vi "Timing-Watchdog.vi"(0 "milliseconds to wait":u32=5000, 7 "Watch":bool) -> ()   [LabVIEW 2020]
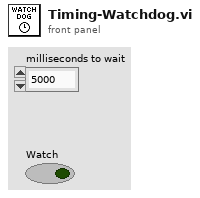
[diagram p1: front panel]
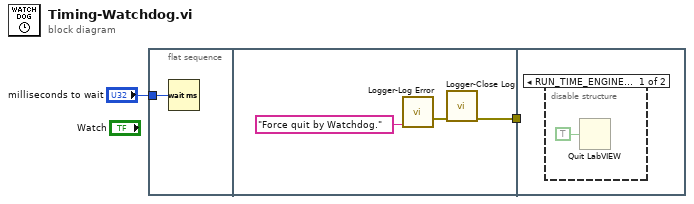
[diagram p0: block diagram]
diagram:
  n1 = flat-sequence {
    tunnel: "milliseconds to wait" -> [w3]
    tunnel: [w6] -> w1
    tunnel: w1 -> [_]
    frame #0 {
      n2 = Wait (ms)(milliseconds to wait=w3) -> ()  [unwired: 1 out]
    }
    frame #1 {
      n3 = call "Logger-Log Error.vi"("Message"="Force quit by Watchdog.") -> ("error out"=w5:errorcluster)  [unwired: 14 in]
      n4 = call "Logger-Close Log.vi"("error in (no error)"=w5) -> ("error out"=w6:errorcluster)  [unwired: 14 in]
    }
    frame #2 {
      n5 = disable-structure shown="RUN_TIME_ENGINE==True, Default" {
        frame condition #0 {
          n6 = Quit LabVIEW(quit? (T)=TRUE) -> ()
        }
        frame condition #1 (active) {
        }
      }
    }
  }
